vi "P3y2v2.vi"(6 "sin sagedus":dbl=1.0, 7 "Puntkide arv":i32=600, 8 "error in (no error)":errorcluster, 9 "cos sagedus":dbl=1.0, 10 "cos amp":dbl=1.0, 11 "sin amp":dbl=1.0) -> (2 "appended array":cluster{i32, i32, dbl[]}[](array[cluster]), 3 "error out":errorcluster)   [LabVIEW 2020]
doc: "Nagu see toimib.... vist Aga muidu teeb meile lahedat arrayd"
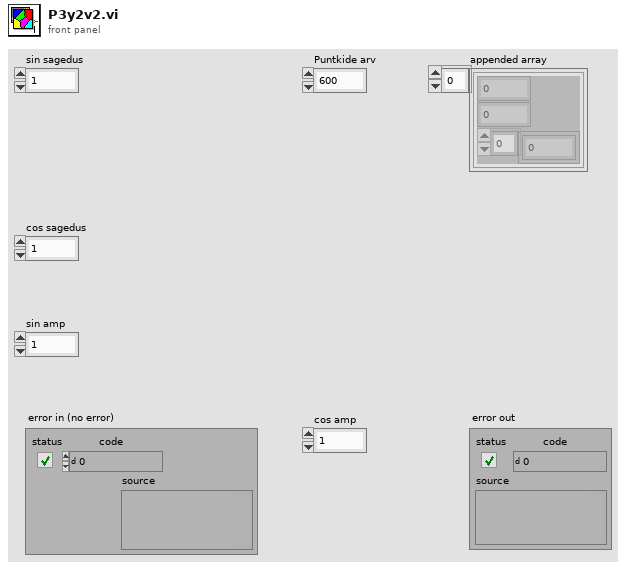
[diagram p1: front panel]
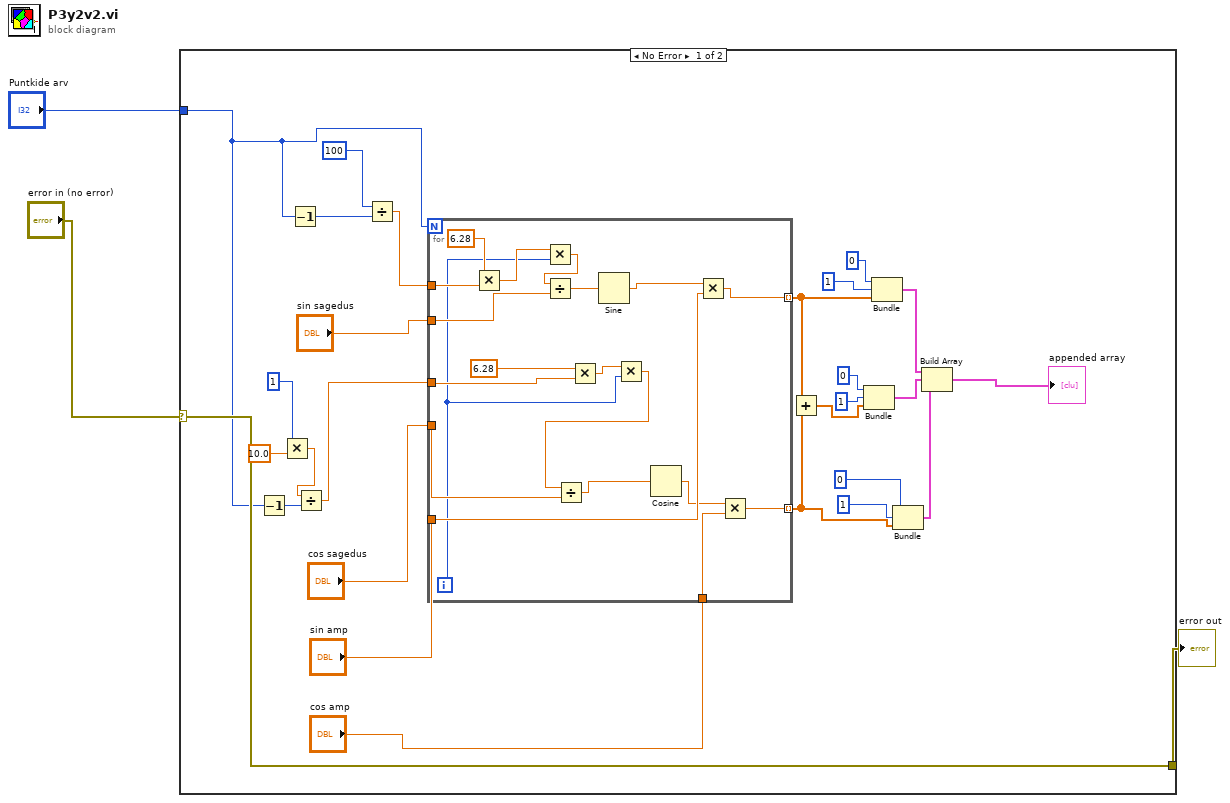
[diagram p0: block diagram]
diagram:
  n1 = case shown="No Error" "error in (no error)" {
    selector: "error in (no error)" -> [w30 w50]
    tunnel: [w30 w50] -> w3
    tunnel: "Puntkide arv" -> [w4 _]
    frame No Error {
      n2 = Decrement(x=w4) -> (x-1=w11:i32)
      n3 = Multiply(x=1, y=10.0) -> (x*y=w6:dbl)
      n4 = Decrement(x=w4) -> (x-1=w13:i32)
      n5 = Divide(x=w6, y=w11) -> (x/y=w9:dbl)
      n6 = Divide(x=100, y=w13) -> (x/y=w10:dbl)
      n7 = for {
        N: w4 -> [_]
        tunnel: "sin sagedus" -> [w49]
        tunnel: "cos sagedus" -> [w48]
        tunnel: "sin amp" -> [w45]
        tunnel: "cos amp" -> [w44]
        tunnel: [w41] -> w19 mode=indexing
        tunnel: [w40] -> w21 mode=indexing
        tunnel: w10 -> [w39]
        tunnel: w9 -> [w35]
        i -> [w32]
        n8 = Multiply(x=6.28, y=w39) -> (x*y=w37:dbl)
        n9 = Multiply(x=w37, y=w32) -> (x*y=w36:dbl)
        n10 = Divide(x=w36, y=w49) -> (x/y=w46:dbl)
        n11 = Multiply(x=6.28, y=w35) -> (x*y=w33:dbl)
        n12 = Sine(x=w46) -> (sin(x)=w43:dbl)
        n13 = Multiply(x=w33, y=w32) -> (x*y=w31:dbl)
        n14 = Divide(x=w31, y=w48) -> (x/y=w47:dbl)
        n15 = Cosine(x=w47) -> (cos(x)=w42:dbl)
        n16 = Multiply(x=w43, y=w45) -> (x*y=w40:dbl)
        n17 = Multiply(x=w42, y=w44) -> (x*y=w41:dbl)
      }
      n18 = Add(x=w21, y=w19) -> (x+y=w20:dbl[])
      n19 = Bundle(0, 1, w20) -> (w15:cluster{i32, i32, dbl[]})  [unwired: 1 in]
      n20 = Bundle(0, 1, w21) -> (w16:cluster{i32, i32, dbl[]})  [unwired: 1 in]
      n21 = Bundle(0, 1, w19) -> (w14:cluster{i32, i32, dbl[]})  [unwired: 1 in]
      n22 = Build Array(w16, w15, w14) -> (→"appended array":cluster{i32, i32, dbl[]}[])
    }
    frame Error {
    }
  }
  "error out" <- w3
